vi "4.4.vi"(2 "use system alert? (T)":bool=TRUE caption="使用系统警报？(T)", 3 "duration (msec)":u32 caption="持续时间（毫秒）", 4 "frequency (Hz)":u32 caption="频率(Hz)", 5 "温度值":dbl) -> ()   [LabVIEW 2017]
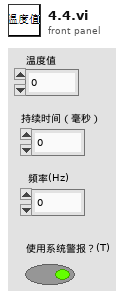
[diagram p1: front panel]
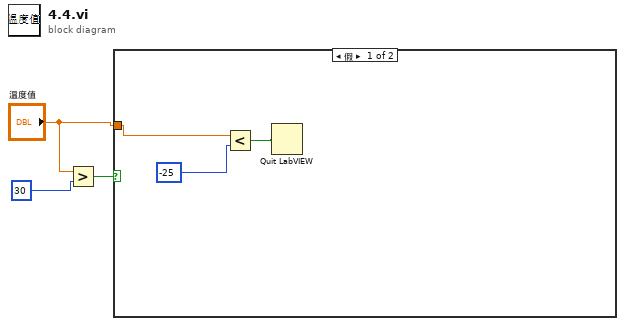
[diagram p0: block diagram]
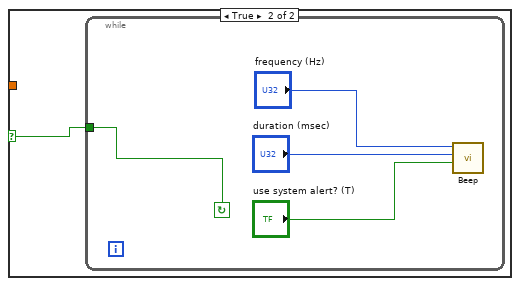
[diagram p2: hidden frame]
diagram:
  n1 = Greater?(x="温度值", y=30) -> (0:w3:bool)
  n2 = case shown="假" w3 {
    selector: w3 -> [_ w7]
    tunnel: "温度值" -> [w4 _]
    frame False {
      n3 = Less?(x=w4, y=-25) -> (x < y?=w6:bool)
      n4 = Quit LabVIEW(quit? (T)=w6) -> ()
    }
    frame True {
      n5 = while {
        tunnel: w7 -> [w11]
        stop <- w11 continue-if-true
        n6 = call <vilib>:"Beep.vi"("use system alert? (T)"="use system alert? (T)", "duration (msec)"="duration (msec)", "frequency (Hz)"="frequency (Hz)") -> ()  [unwired: 9 in]
      }
    }
  }
